vi "Pop Up.vi"(11 "Pop Up in":refnum<class "Pop Up.lvclass">) -> (3 "Pop Up out":refnum<class "Pop Up.lvclass">)   [LabVIEW 2021, in "jettl Msg Pop Up.lvlib" / "Pop Up.lvclass"]
uses:
  Pop Up.lvclass
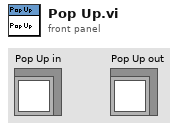
[diagram p1: front panel]
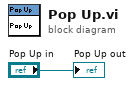
[diagram p0: block diagram]
diagram:
  "Pop Up out" <- "Pop Up in"
